vi "PPMS2_Parent.vi"() -> ()   [LabVIEW 2013]
uses:
  <vilib>/lvdsc/historical/Open Trace (Numeric).vi
  <vilib>/lvdsc/historical/Write Trace (Numeric).vi
  <vilib>/lvdsc/NI_DSC.lvlib
panel:
  in  "pattern":string="ppms2log*.dat"
  in  "Folder Path In":path=path "\\\\PPMS2\\Data/PPMS Log"
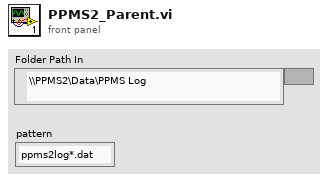
[diagram p1: front panel]
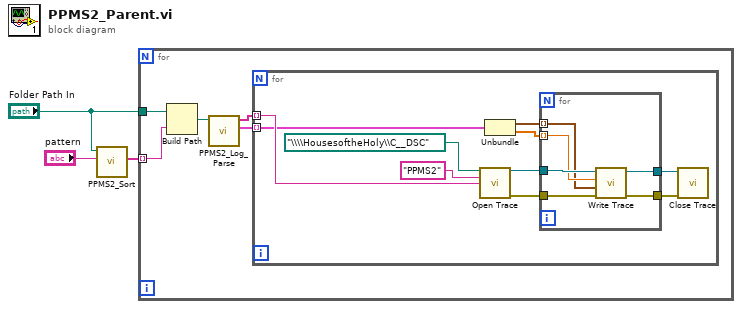
[diagram p0: block diagram]
diagram:
  n1 = call "PPMS2_Sort.vi"("pattern"="pattern", "directory path"="Folder Path In") -> ("Array"=w1:string[])  [unwired: 7 in]
  n2 = for {
    tunnel: w1 -> [w8] mode=indexing
    tunnel: "Folder Path In" -> [w7]
    n3 = Build Path(base path=w7, name or relative path=w8) -> (appended path=w6:path)
    n4 = call "PPMS2_Log_Parse.vi"("file path (dialog if empty)"=w6) -> ("XY Graph"=w4:cluster{timestamp[], dbl[]}[], "Array"=w5:string[])  [unwired: 9 in]
    n5 = for {
      tunnel: w5 -> [w12] mode=indexing
      tunnel: w4 -> [w11] mode=indexing
      n6 = call-poly <vilib>:"Open Trace.vi"("database URL"=path "\\\\HousesoftheHoly\\C__DSC", "process name"="PPMS2", "trace name"=w12) -> ("trace reference"=w14:refnum<k1>, "error out"=w13:errorcluster)  [unwired: 10 in, 1 out]
      n7 = Unbundle(w11) -> (w10:timestamp[], w9:dbl[])
      n8 = for {
        tunnel: [w24] -> w16
        tunnel: [w23] -> w15
        tunnel: w14 -> [w22]
        tunnel: w13 -> [w21]
        tunnel: w10 -> [w19] mode=indexing
        tunnel: w9 -> [w20] mode=indexing
        n9 = call-poly <vilib>:"Write Trace.vi"("error in (no error)"=w21, "timestamp (now)"=w19, "value"=w20, "trace ref"=w22) -> ("error out"=w24:errorcluster, "trace ref out"=w23:refnum<k1>)  [unwired: 6 in]
      }
      n10 = call <vilib>:"Close Trace.vi"("error in (no error)"=w16, "trace reference"=w15) -> ()  [unwired: 9 in, 1 out]
    }
  }
